vi "pop_stack.vi"(1 "pilha input":T1[](array[typedef])) -> (8 "pilha output":T1[](array[typedef]))   [LabVIEW 2016]
uses:
  segment.ctl
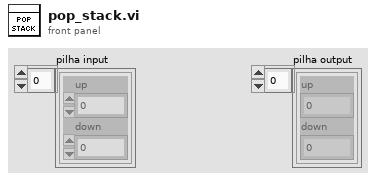
[diagram p1: front panel]
types:
  T1 = typedef "segment.ctl" = cluster{"up":dbl, "down":dbl}
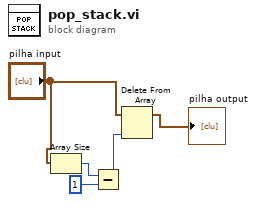
[diagram p0: block diagram]
diagram:
  n1 = Array Size(array="pilha input") -> (size(s)=w3:i32)
  n2 = Subtract(x=w3, y=1) -> (x-y=w1:i32)
  n3 = Delete From Array(array="pilha input", index=w1) -> (array with subset deleted=→"pilha output":T1[])  [unwired: 1 in, 1 out]
